vi "SPC_init_buf_stream.vi"(4 "Start01_offs ( for DPC modules)":u32, 5 "Stream Type":i16=1 max=1536 step=1 format="%x", 6 "MT clock ( 0.1 ns units)":i32, 7 "FIFO Type":T2=7 items=["48 bits SPC-6x0"=2, "32 bits SPC-6x0"=3, "32 bits SPC-130"=4, "32 bits SPC-830"=5, "32 bits SPC-140"=6, "32 bits SPC-150\\160\\180"=7, "32 bits DPC-230"=8, "32 bits FIFO_IMAGE"=9, "FIFO_D590"=10, "FIFO_TDC"=11, "FIFO_TDC_ABS"=12], 8 "Error In":errorcluster, 9 "What to Read":T1, 10 "Module No":i16, 11 "DLL Path":path) -> (0 "Error Out":errorcluster, 1 "Stream Handle":i16=-1, 2 "Module No":i16, 3 "DLL Path":path)   [LabVIEW 2017]
doc: "The procedure is needed to initiate the process of extracting photons from a stream of photons placed into PC memory buffers previously 'buffered' stream. \nTo get input parameters needed to call SPC_init_buf_stream (fifo_type, stream_type, \nmt_clock) call SPC_get_fifo_init_vars function, when you are ready to start the FIFO \nmeasurement.\nIf the photons are taken from .spc files, input parameters should be taken from .spc file header (1st word).\nSet bit 9 of 'stream_type' if the file contains markers (was created in FIFO_IMG mode or FIFO mode with enabled markers).\nBuffers are allocated/reallocated automatically while adding photons to the stream. \nThe buffers can be freed in two ways depending on an option FREE_BUF_STREAM ( bit 13 \nin 'stream_type' parameter). \nIf bit 13 is not set, the buffers are freed when the stream is closed (SPCM_close_phot_stream).\nIf bit 13 is set, the buffer will be freed, when, during SPC_get_photons_from_stream call, all \nphotons from the current buffer are extracted.\nAfter this it will be not possible to use the buffer again, for example to get data from it using \nSPC_get_buffer_from_stream function.\nFREE_BUF_STREAM option is recommended for long measurements with lots of data read from FIFO, which could make buffers allocated space very (too) big.\nIf the photons rate or measurement time is not very big/long, buffers can stay allocated and another extract action can be started (with different start/stop condition) or buffers contents can be stored in .spc file.\nUser can add photons to the stream buffers by using function:\nSPC_add_data_to_stream - photons are taken from the buffer ( input buffer can be filled from .spc file)\nSPC_read_fifo_to_stream - photons are read from FIFO during running FIFO measurement. \nAdding photons to the stream or extracting photons can be done also during running measurement. During extracting or adding photons the stream is locked. Only one thread can access the thread safe stream at a time. If a thread requests the access to stream resources while another has it, the second thread waits in this function until the first thread releases the \nstream.\nUse function SPC_get_photons_from_stream to extract photons information from the stream buffers.\n'fifo_type parameter defines the format of the photons data in the stream. It depends mainly on the SPC module type which was used during the measurement. Possible 'fifo_type' values are defined in the spcm_def.h file.\n'what_to_read' parameter defines which entries will be extracted from the stream. \nIn most cases only bit 0 will be set (valid photons). For streams containing also markers -\nmarkers 0-3 (pixel, line, frame) can also be extracted (bits 2-5).\nIf the stream is successfully initialised, the procedure creates internal DLL PhotStreamInfo structure and returns the handle to the stream (positive value). Use this handle as an input parameter to the other extraction functions (SPC_close_phot_stream, SPC_get_phot_stream_info, SPC_get_photons_from_stream and so on ).\nMax 8 streams can be initialised by the SPCM DLL.\nUse SPC_get_phot_stream_info to get the current state of the stream and SPC_get_photons_from_stream to extract subsequent photons from the stream.\nUsing SPC_stream_start_condition and SPC_stream_stop_condition user can define start/stop condition of extracting photons, which can be specific macro time and/or occurrence of markers or routing channels.\nAs long as stream buffers are not freed user can call SPC_reset_stream and then extract photons again with another start/stop condition.\nAfter extracting photons stream should be closed using SPC_close_phot_stream function.\nSee use_spcm.c file for the extraction example.\n\nstream_type \n bit 0 has no special meaning for buffered streams, is set to 1\n bits 1,2,8 = 0, used only for DPC-230 FIFO data\n bit 9 = 1 - stream contains marker entries ( FIFO_IMG mode )\n bit 10 = 1 - stream contains raw data ( diagnostics only )\n bit 12 = 1 - indicates buffered stream type\n bit 13 = 1 - stream buffer freed automatically after extracting photons from it\n = 0 . stream buffer freed using SPC_close_phot_stream\nwhat_to_read defines which entries will be extracted \n bit 0 = 1 read valid photons, \n bit 1 = 1 read invalid photons,\n bit 2 = 1 read markers 0 (pixel), \n bit 3 = 1 read markers 1 (line),\n bit 4 = 1 read markers 2 (frame), \n bit 5 = 1 read markers 3\n\ninfo@becker-hickl.com"
uses:
  SPC_Controls/Fifo_Type.ctl
  SPC_Controls/WhatToRead.ctl
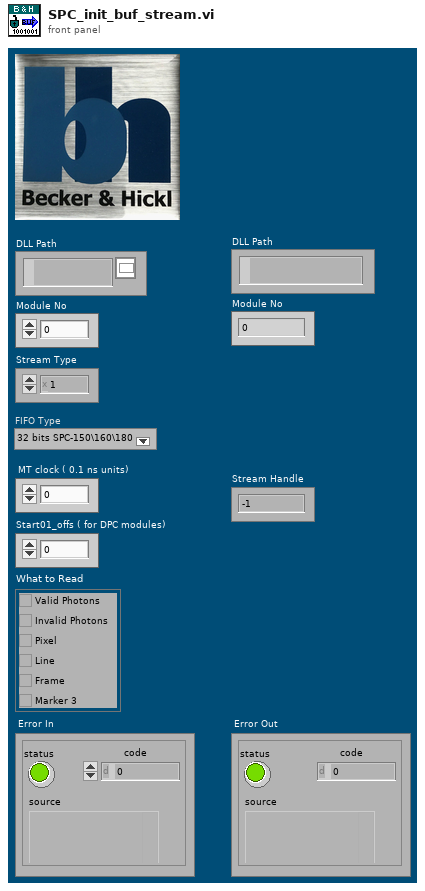
[diagram p1: front panel]
types:
  T1 = typedef "WhatToRead.ctl" = cluster{"Valid Photons":bool, "Invalid Photons":bool, "Pixel":bool, "Line":bool, "Frame":bool, "Marker 3":bool}
  T2 = typedef "Fifo_Type.ctl" = i16
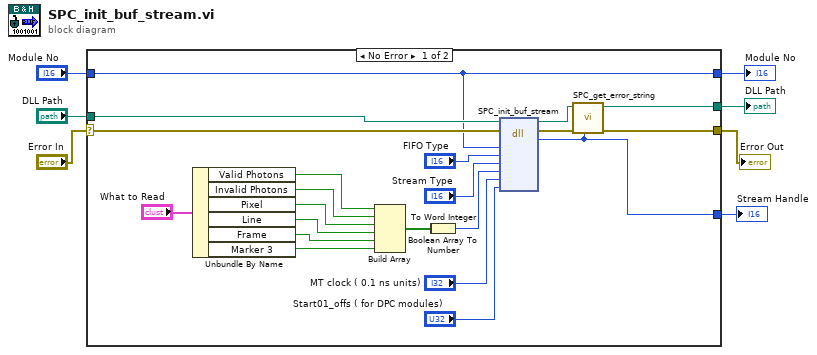
[diagram p0: block diagram]
diagram:
  n1 = case shown="No Error" "Error In" {
    selector: "Error In" -> [w26 w32]
    tunnel: [w23 w32] -> w6
    tunnel: "DLL Path" -> [w25 w31]
    tunnel: [w21 w31] -> w4
    tunnel: "Module No" -> [w8 w30]
    tunnel: [w8 w30] -> w2
    tunnel: [w9 _] -> w1
    frame No Error {
      n2 = Unbundle By Name("What to Read") -> ("Valid Photons"=w19:bool, "Invalid Photons"=w18:bool, "Pixel"=w17:bool, "Line"=w16:bool, "Frame"=w15:bool, "Marker 3"=w14:bool)
      n3 = Build Array(w19, w18, w17, w16, w15, w14) -> (w13:bool[])
      n4 = Boolean Array To Number(Boolean array=w13) -> (number=w12:u32)
      n5 = To Word Integer(number=w12) -> (16bit integer=w11:i16)
      n6 = dll-call lib="D:/spcm/lib/lab_view/lv10.0/spcm32.dll" fn="SPC_init_buf_stream"(path in=w25, error in=w26, "mod_no"=w8, "fifo_type"="FIFO Type", "stream_type"="Stream Type", "what_to_read"=w11, "mt_clock"="MT clock ( 0.1 ns units)", "start01_offs"="Start01_offs ( for DPC modules)") -> (path out=w22:path, error out=w24:errorcluster, "return type"=w9:i16)  [unwired: 7 in]
      n7 = call "SPC_get_error_string.vi"("ErrorID"=w9, "Error In"=w24, "DLL Path"=w22) -> ("Error Out"=w23:errorcluster, "DLL Path"=w21:path)  [unwired: 6 in, 1 out]
    }
    frame Error {
    }
  }
  "Error Out" <- w6
  "DLL Path" <- w4
  "Module No" <- w2
  "Stream Handle" <- w1
